vi "FollowBallAfterPassSkill.vi"(6 "ReceiverPosition":dbl[](array[numeric]), 8 "error in (no error)":errorcluster, 9 "Ball":refnum<class "Ball.lvclass">, 10 "Robot in":refnum<class "Robot.lvclass">, 11 "FollowBallAfterPassSkill in":refnum<class "FollowBallAfterPassSkill.lvclass">) -> (0 "error out":errorcluster, 2 "Robot out":refnum<class "Robot.lvclass">, 3 "FollowBallAfterPassSkill out":refnum<class "FollowBallAfterPassSkill.lvclass">)   [LabVIEW 2023, in "FollowBallAfterPassSkill.lvclass"]
uses:
  FollowBallAfterPassSkill.lvclass
  Robot_class/Robot.lvclass
  Ball_class/Ball.lvclass
  C:/Users/lucio/Desktop/roboime/SSL_AI/Object_class/Object.lvclass
  Object_class/Object.lvclass/Object.ctl
  Ball_class/Ball.lvclass/Ball.ctl
  Robot_class/Robot.lvclass/Robot.ctl
  HaltSkill_class/HaltSkill.lvclass
  <vilib>/Analysis/baseanly.llb/Unit Vector (DBL).vi
  Robot_class/Write dest_x.vi
  Robot_class/Write dest_y.vi
  Robot_class/Write dest_orientation.vi
  Object_class/Read position(x,y).vi
  Ball_class/Read v_x.vi
  Ball_class/Read v_y.vi
  <vilib>/Analysis/NI_AALBase.lvlib
  Utilities_class/Utilities.lvclass
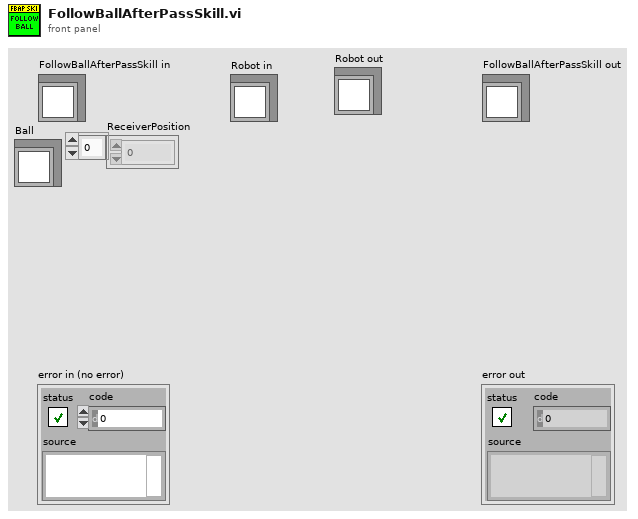
[diagram p1: front panel]
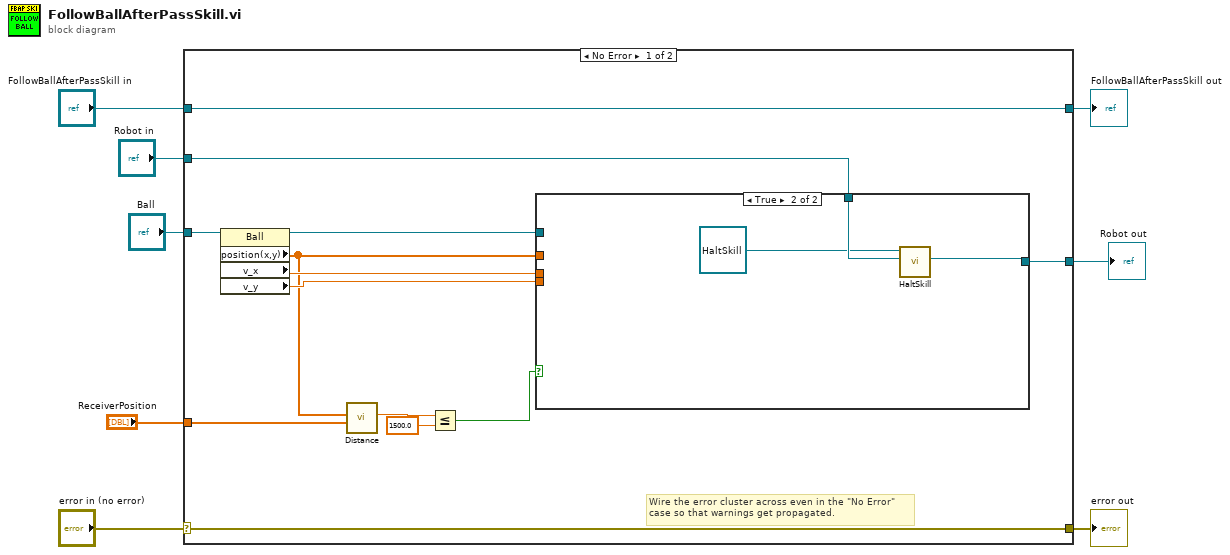
[diagram p0: block diagram]
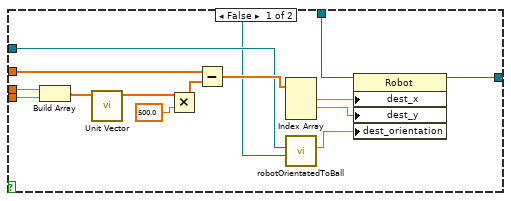
[diagram p2: hidden frame]
diagram:
  n1 = case shown="No Error" "error in (no error)" {
    selector: "error in (no error)" -> [w20 w40]
    tunnel: [w20 w40] -> w7
    tunnel: [w21 w39] -> w5
    tunnel: "FollowBallAfterPassSkill in" -> [w21 w39]
    tunnel: "Ball" -> [w19 _]
    tunnel: "Robot in" -> [w15 _]
    tunnel: [w14 _] -> w2
    tunnel: "ReceiverPosition" -> [w13 _]
    frame No Error {
      # "Wire the error cluster across even in the \"No Error\"\ncase so that warnings get propagated."
      n2 = property class="Ball"(reference=w19) -> (reference out=w16:refnum<class "Ball.lvclass">, "position(x,y)"=w12:dbl[], "v_x"=w18:dbl, "v_y"=w17:dbl)  [unwired: 1 in, 1 out]
      n3 = call "Distance.vi"("P1"=w13, "P2"=w12) -> ("Distance"=w11:dbl)  [unwired: 7 in, 2 out]
      n4 = Less Or Equal?(x=w11, y=1500.0) -> (x <= y?=w9:bool)
      n5 = case shown="True" w9 {
        tunnel: w18 -> [w35 _]
        tunnel: w17 -> [w34 _]
        tunnel: w16 -> [w25 _]
        tunnel: w15 -> [w24 w37]
        tunnel: [w23 w38] -> w14
        tunnel: w12 -> [w22 _]
        frame False {
          n6 = Build Array(w35, w34) -> (w33:dbl[])
          n7 = call-poly <vilib>:"Unit Vector.vi"("Input Vector"=w33) -> ("Unit Vector"=w32:dbl[])  [unwired: 8 in, 2 out]
          n8 = Multiply(x=w32, y=500.0) -> (x*y=w31:dbl[])
          n9 = Subtract(x=w22, y=w31) -> (x-y=w29:dbl[])
          n10 = Index Array(array=w29) -> (element #1=w28:dbl, element #2=w27:dbl)  [unwired: 3 in, 1 out]
          n11 = call "robotOrientatedToBall.vi"("Robot"=w24, "BallRef"=w25) -> ("Orientation"=w26:dbl)  [unwired: 7 in, 2 out]
          n12 = property class="Robot"(reference=w24, "dest_x"=w28, "dest_y"=w27, "dest_orientation"=w26) -> (reference out=w23:refnum<class "Robot.lvclass">)  [unwired: 1 in, 1 out]
        }
        frame True {
          n13 = call-dynamic "HaltSkill.vi"("Robot"=w37, "HaltSkill in"=refnum<class "HaltSkill.lvclass"> refnum) -> ("Robot out"=w38:refnum<class "Robot.lvclass">)  [unwired: 7 in, 2 out]
        }
      }
    }
    frame Error {
    }
  }
  "error out" <- w7
  "FollowBallAfterPassSkill out" <- w5
  "Robot out" <- w2
